vi "Write Element.vi"(8 "error in (no error)":errorcluster, 10 "Element.lvclass":refnum<class "Abs_Type.lvclass">, 11 "Array Element 1D in":refnum<class "Vector of Elements.lvclass">) -> (0 "error out":errorcluster, 3 "Array Element 1D out":refnum<class "Vector of Elements.lvclass">)   [LabVIEW 2019, in "Vector of Elements.lvclass"]
uses:
  Vector of Elements.lvclass
  Type/Abs_Type.lvclass
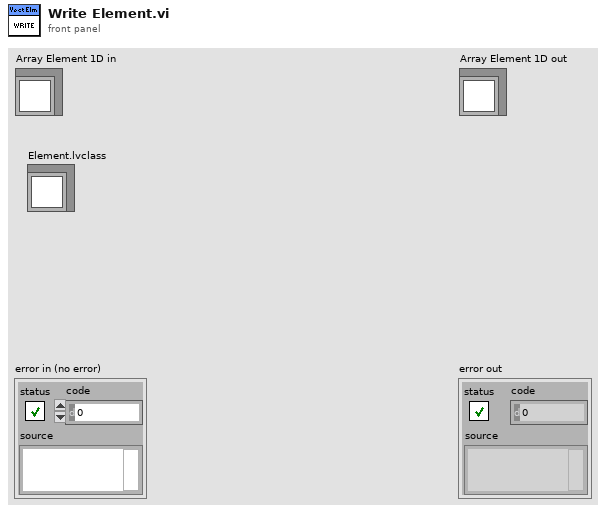
[diagram p1: front panel]
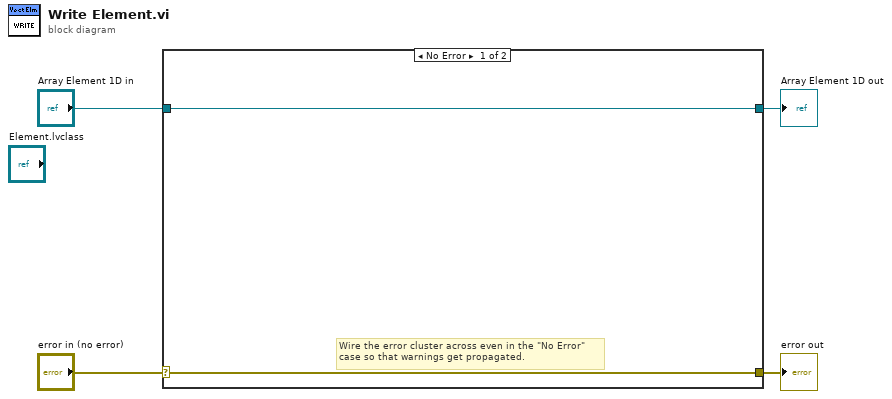
[diagram p0: block diagram]
diagram:
  n1 = case shown="No Error" "error in (no error)" {
    selector: "error in (no error)" -> [w5 w8]
    tunnel: [w5 w8] -> w3
    tunnel: [w6 w7] -> w1
    tunnel: "Array Element 1D in" -> [w6 w7]
    frame No Error {
      # "Wire the error cluster across even in the \"No Error\"\ncase so that warnings get propagated."
    }
    frame Error {
    }
  }
  "error out" <- w3
  "Array Element 1D out" <- w1
